vi "get controls from tab.vi"(11 "TabControl in":refnum<vi>) -> (2 "appended array":refnum<vi>[](array[refnum]), 3 "Array 3":string[](array[string]))   [LabVIEW 2011]
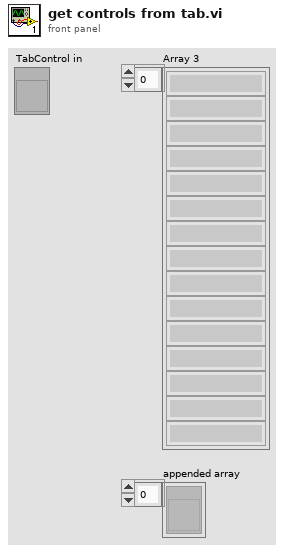
[diagram p1: front panel]
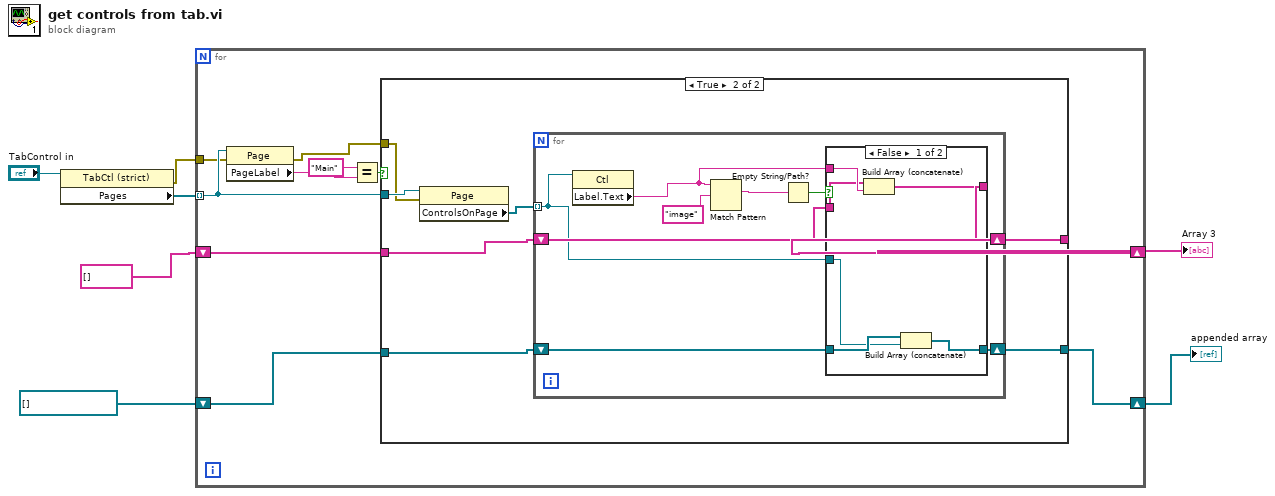
[diagram p0: block diagram]
diagram:
  n1 = property on="Property Node" class="TabCtl (strict)"(reference="TabControl in") -> (error out=w3:errorcluster, "Pages"=w2:refnum<vi>[])  [unwired: 1 in, 1 out]
  n2 = for {
    tunnel: w2 -> [w17] mode=indexing
    tunnel: w3 -> [w13]
    shift-right: [w10] -> w5
    shift-left: string[] [] ("Array 3") -> [w11]
    shift-right: [w8] -> w7
    shift-left: refnum<vi>[] [] ("appended array") -> [w9]
    n3 = property class="Page"(reference=w17, error in=w13) -> (error out=w12:errorcluster, "PageLabel"=w15:string)  [unwired: 1 out]
    n4 = Equal?(x="Main", y=w15) -> (x = y?=w16:bool)
    n5 = case shown="True" w16 {
      tunnel: w17 -> [_ w26]
      tunnel: w12 -> [_ w25]
      tunnel: w11 -> [w19 w23]
      tunnel: [w19 w22] -> w10
      tunnel: w9 -> [w18 w21]
      tunnel: [w18 w20] -> w8
      frame False {
      }
      frame True {
        n6 = property class="Page"(reference=w26, error in=w25) -> ("ControlsOnPage"=w24:refnum<vi>[])  [unwired: 2 out]
        n7 = for {
          tunnel: w24 -> [w27] mode=indexing
          shift-right: [w30] -> w22
          shift-left: w23 -> [w31]
          shift-right: [w28] -> w20
          shift-left: w21 -> [w29]
          n8 = property class="Ctl"(reference=w27) -> ("Label.Text"=w32:string)  [unwired: 1 in, 2 out]
          n9 = Match Pattern(string=w32, regular expression="image") -> (match substring=w34:string)  [unwired: 1 in, 3 out]
          n10 = Empty String/Path?(string/path=w34) -> (empty?=w33:bool)
          n11 = case shown="False" w33 {
            tunnel: w32 -> [w41 _]
            tunnel: w31 -> [w40 w43]
            tunnel: [w39 w43] -> w30
            tunnel: w27 -> [w37 _]
            tunnel: w29 -> [w38 w42]
            tunnel: [w36 w42] -> w28
            frame False {
              n12 = Build Array (concatenate)(w40, w41) -> (w39:string[])
              n13 = Build Array (concatenate)(w38, w37) -> (w36:refnum<vi>[])
            }
            frame True {
            }
          }
        }
      }
    }
  }
  "Array 3" <- w5
  "appended array" <- w7
